vi "DQ_test.vi"() -> ()   [LabVIEW 2015]
uses:
  <vilib>/Analysis/NI_AALBase.lvlib
  AlphaBetaAndDQ_variants/DQtoABC_PowerInvariant_src.vi
  AlphaBetaAndDQ_variants/DQtoABC_noSine_PowerInvariant_src.vi
  AlphaBetaAndDQ_variants/ABCtoDQ_3PhasePowerInvariant_src.vi
  AlphaBetaAndDQ_variants/ABCtoDQ_noSine_2PhasePowerInvariant_src.vi
  AlphaBetaAndDQ_variants/ABCtoDQ_noSine_3PhasePowerInvariant_src.vi
  AlphaBetaAndDQ_variants/ABCtoDQ_2PhasePowerInvariant_src.vi
  AlphaBetaAndDQ_variants/ABCtoDQ_2PhaseUnitaryMagnitude_src.vi
  AlphaBetaAndDQ_variants/DQtoABC_UnitaryMagnitude_src.vi
  AlphaBetaAndDQ_variants/ABCtoDQ_3PhaseUnitaryMagnitude_src.vi
  AlphaBetaAndDQ_variants/ABCtoDQ_noSine_2PhaseUnitaryMagnitude_src.vi
  AlphaBetaAndDQ_variants/DQtoABC_noSine_UnitaryMagnitude_src.vi
  AlphaBetaAndDQ_variants/ABCtoDQ_noSine_3PhaseUnitaryMagnitude_src.vi
  <vilib>/addons/E-Motor Simulation/Utility/NI_EMSim_Utility.lvlib
panel:
  out "2 phase UM error (no sine) stddev":dbl format="%0.2f"
  out "2 phase UM (no Sine) error max":dbl
  out "2 phase UM (no sine) error mean":dbl format="%0.2f"
  out "3phase UM (no sine)error stddev":dbl format="%0.2f"
  out "3 phase UM (no sine) error max":dbl
  out "3 phase UM (no sine) error mean":dbl format="%0.2f"
  out "3 phase UM error stddev":dbl format="%0.2f"
  out "2 phase UM error stddev":dbl format="%0.2f"
  out "3 phase UM error max":dbl
  out "3 phase UM error mean":dbl format="%0.2f"
  out "2 phase UM error max":dbl
  out "2 phase UM error mean":dbl format="%0.2f"
  out "transposed array":sgl[][](graph)
  out "2 phase PI (no sine) error mean":dbl format="%0.2f"
  out "2 phase PI (no Sine) error max":dbl
  out "2 phase PI error (no sine) stddev":dbl format="%0.2f"
  out "3 phase PI (no sine) error mean":dbl format="%0.2f"
  out "3 phase PI (no sine) error max":dbl
  out "3phase PI (no sine)error stddev":dbl format="%0.2f"
  out "3 phase PI error stddev":dbl format="%0.2f"
  out "2 phase PI error stddev":dbl format="%0.2f"
  in  "Imbalance (percent)":dbl
  in  "GridImbalance":bool
  in  "InjectAdditiveNoise":bool
  in  "Noise Magnitude (percent)":dbl
  in  "Magnitude":dbl=1.0
  out "3 phase PI error max":dbl
  out "3 phase PI error mean":dbl format="%0.2f"
  out "2 phase PI error max":dbl
  out "2 phase PI error mean":dbl format="%0.2f"
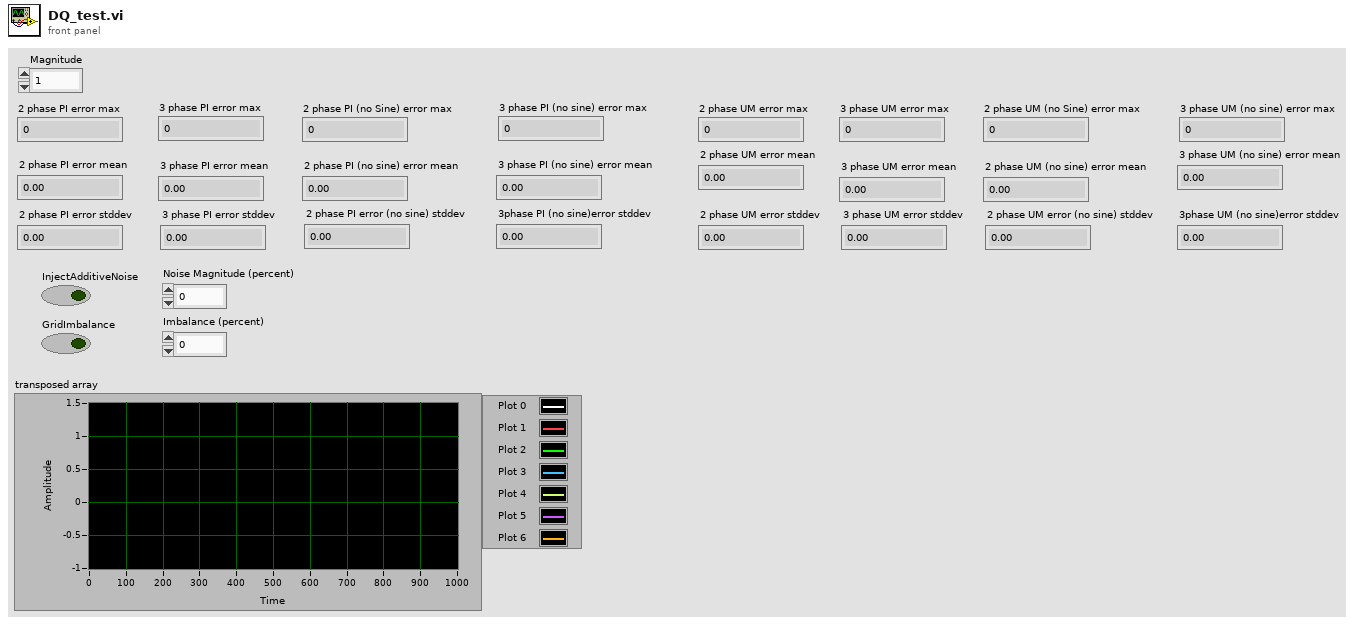
[diagram p1: front panel]
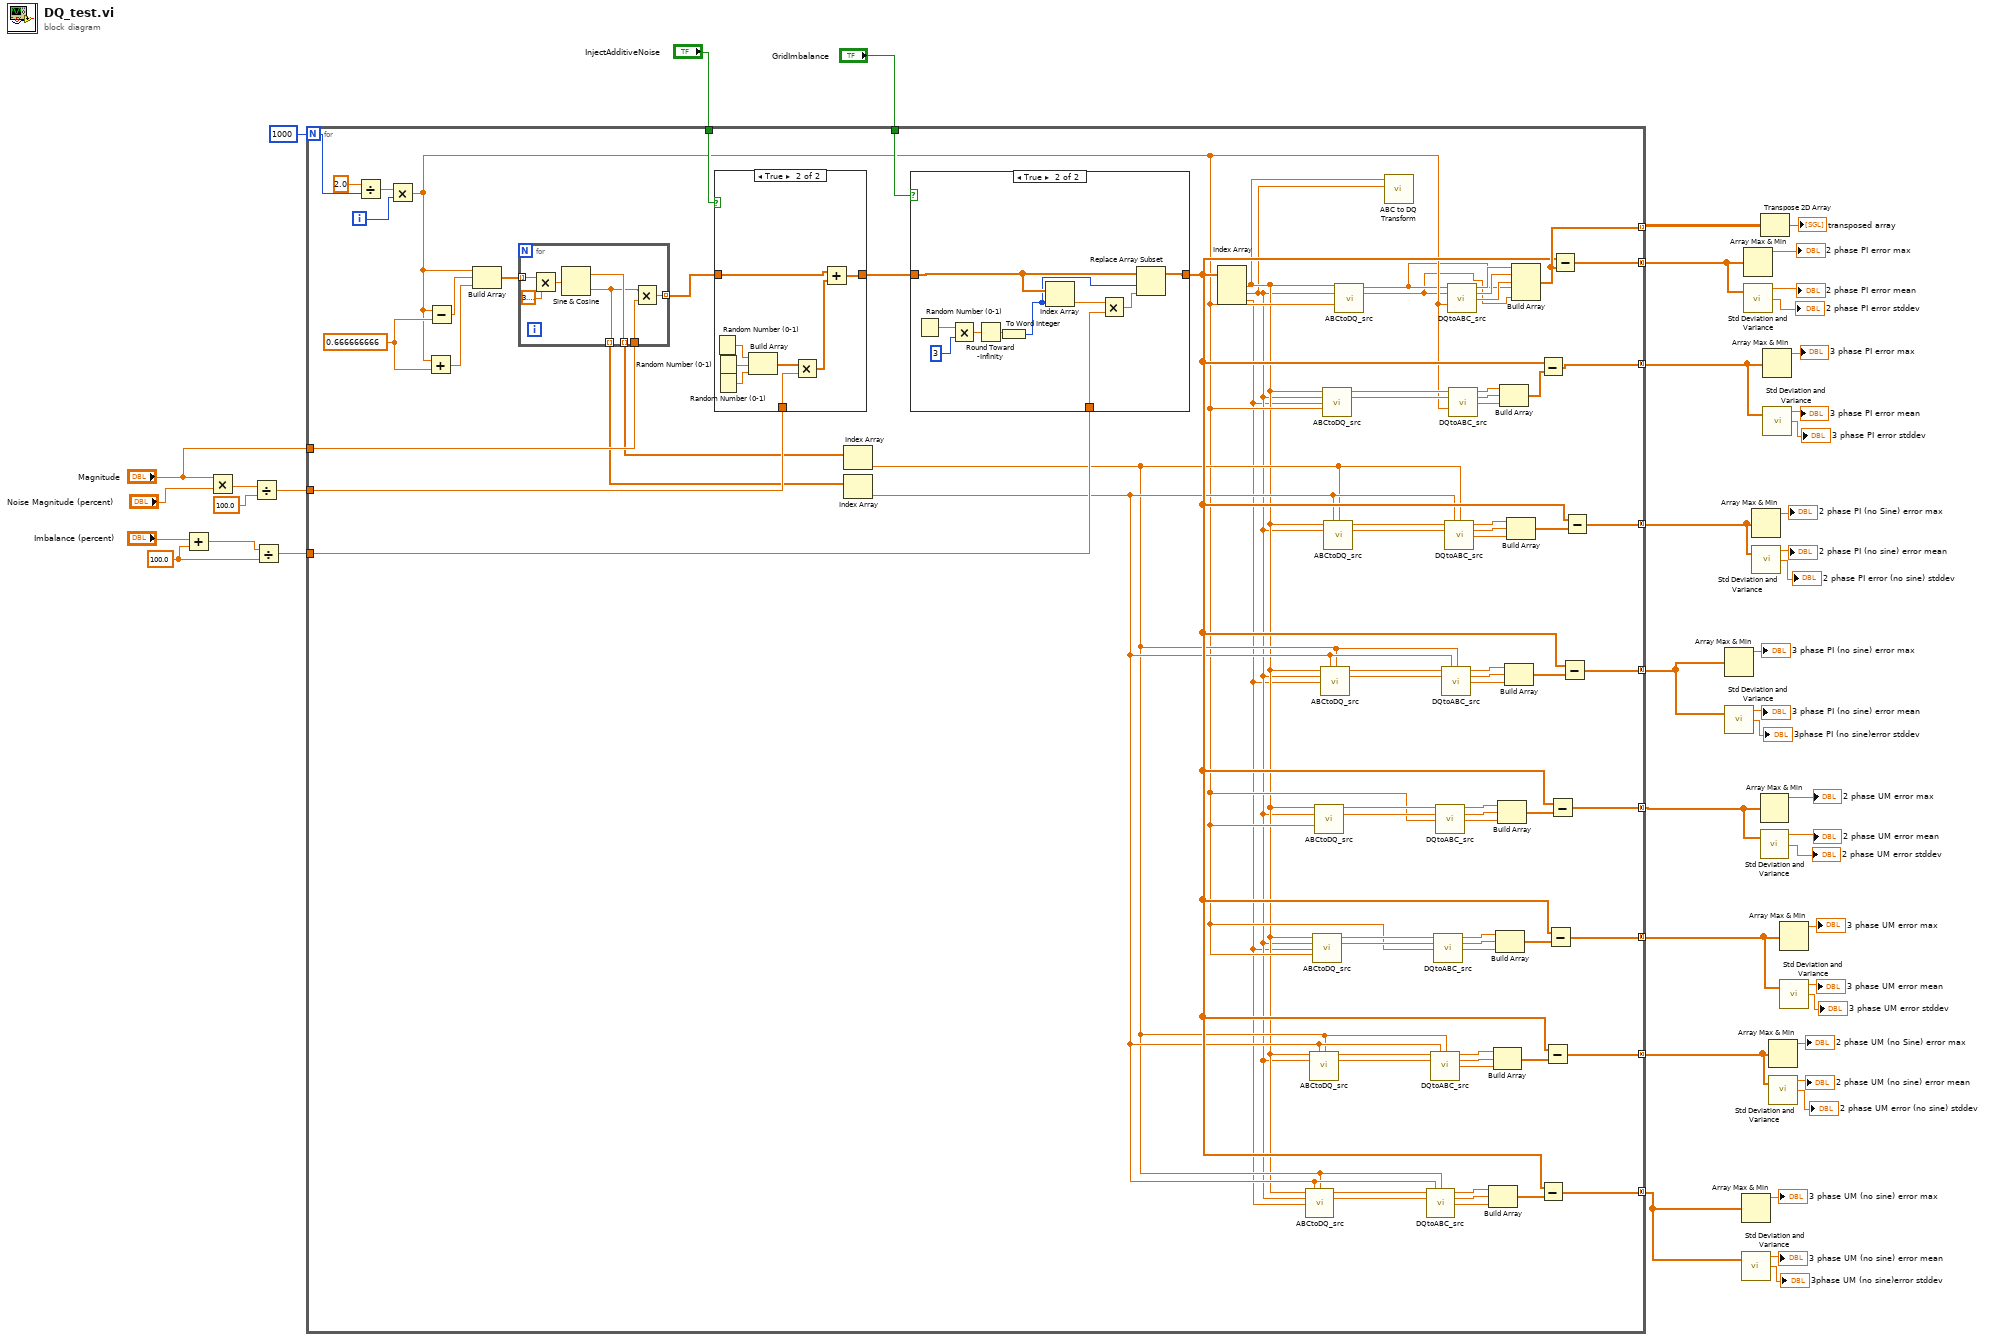
[diagram p0: block diagram]
diagram:
  w31 = 100.0 ("y")
  n1 = Add(x="Imbalance (percent)", y=w31) -> (x+y=w32:dbl)
  n2 = Multiply(x="Magnitude", y="Noise Magnitude (percent)") -> (x*y=w39:dbl)
  n3 = Divide(x=w39, y=100.0) -> (x/y=w36:dbl)
  n4 = Divide(x=w32, y=w31) -> (x/y=w30:dbl)
  n5 = for {
    N: 1000 -> [w115]
    tunnel: [w112] -> w43 mode=concatenating
    tunnel: [w95] -> w19 mode=concatenating
    tunnel: "Magnitude" -> [w122]
    tunnel: w36 -> [w121]
    tunnel: "InjectAdditiveNoise" -> [w120]
    tunnel: "GridImbalance" -> [w119]
    tunnel: w30 -> [w117]
    tunnel: [w102] -> w27 mode=concatenating
    tunnel: [w88] -> w20 mode=concatenating
    tunnel: [w85] -> w17 mode=indexing
    tunnel: [w71] -> w4 mode=concatenating
    tunnel: [w55] -> w3 mode=concatenating
    tunnel: [w54] -> w2 mode=concatenating
    tunnel: [w53] -> w1 mode=concatenating
    i -> [w113]
    w126 = 0.666666666
    n6 = Divide(x=2.0, y=w115) -> (x/y=w114:dbl)
    n7 = Multiply(x=w114, y=w113) -> (x*y=w52:dbl)
    n8 = Add(x=w52, y=w126) -> (x+y=w124:dbl)
    n9 = Subtract(x=w52, y=w126) -> (x-y=w123:dbl)
    n10 = Build Array(w52, w123, w124) -> (w125:dbl[])
    n11 = for {
      tunnel: w125 -> [w153] mode=indexing
      tunnel: [w151] -> w84 mode=indexing
      tunnel: w122 -> [w150]
      tunnel: [w148] -> w87 mode=indexing
      tunnel: [w147] -> w86 mode=indexing
      n12 = Multiply(x=w153, y=3.141592653589793) -> (x*y=w149:dbl)
      n13 = Sine & Cosine(0:w149) -> (1:w148:dbl, 2:w147:dbl)
      n14 = Multiply(x=w147, y=w150) -> (x*y=w151:dbl)
    }
    n15 = case shown="True" w120 {
      tunnel: w84 -> [w138 w140]
      tunnel: [w138 w139] -> w118
      tunnel: w121 -> [_ w142]
      frame False {
      }
      frame True {
        n16 = Random Number (0-1)() -> (number: 0 to 1=w145:dbl)
        n17 = Random Number (0-1)() -> (number: 0 to 1=w146:dbl)
        n18 = Random Number (0-1)() -> (number: 0 to 1=w144:dbl)
        n19 = Build Array(w145, w146, w144) -> (w143:dbl[])
        n20 = Multiply(x=w143, y=w142) -> (x*y=w141:dbl[])
        n21 = Add(x=w140, y=w141) -> (x+y=w139:dbl[])
      }
    }
    n22 = Index Array(array=w87) -> (element=w56:dbl)  [unwired: 1 in]
    n23 = Index Array(array=w86) -> (element=w57:dbl)  [unwired: 1 in]
    n24 = case shown="True" w119 {
      tunnel: w118 -> [w127 w131]
      tunnel: w117 -> [_ w132]
      tunnel: [w127 w129] -> w58
      frame False {
      }
      frame True {
        n25 = Random Number (0-1)() -> (number: 0 to 1=w137:dbl)
        n26 = Multiply(x=w137, y=3) -> (x*y=w135:dbl)
        n27 = Round Toward -Infinity(1:w135) -> (0:w134:dbl)
        n28 = To Word Integer(number=w134) -> (16bit integer=w128:i16)
        n29 = Index Array(array=w131, index=w128) -> (element=w133:dbl)
        n30 = Multiply(x=w133, y=w132) -> (x*y=w130:dbl)
        n31 = Replace Array Subset(array=w131, new element=w130, index=w128) -> (w129:dbl[])
      }
    }
    n32 = Index Array(array=w58) -> (element #1=w49:dbl, element #2=w48:dbl, element #3=w47:dbl)  [unwired: 3 in]
    n33 = call-poly "ABCtoDQ_src.vi"("A"=w49, "cosx"=w57, "sinx"=w56, "B"=w48, "C"=w47) -> ("direct"=w64:sgl, "quadrature"=w63:sgl)  [unwired: 7 in, 2 out]
    n34 = call-poly "ABCtoDQ_src.vi"("A"=w49, "cosx"=w57, "sinx"=w56, "B"=w48) -> ("direct"=w65:sgl, "quadrature"=w66:sgl)  [unwired: 8 in, 2 out]
    n35 = call-poly "ABCtoDQ_src.vi"("A"=w49, "B"=w48, "C"=w47, "Theta"=w52) -> ("direct"=w77:sgl, "quadrature"=w76:sgl)  [unwired: 6 in, 4 out]
    n36 = call-poly "ABCtoDQ_src.vi"("A"=w49, "B"=w48, "Theta"=w52) -> ("direct"=w78:sgl, "quadrature"=w79:sgl)  [unwired: 7 in, 4 out]
    n37 = call-poly "ABCtoDQ_src.vi"("A"=w49, "cosx"=w57, "sinx"=w56, "B"=w48, "C"=w47) -> ("direct"=w94:sgl, "quadrature"=w93:sgl)  [unwired: 7 in, 2 out]
    n38 = call-poly "ABCtoDQ_src.vi"("A"=w49, "B"=w48, "C"=w47, "Theta"=w52) -> ("direct"=w107:sgl, "quadrature"=w108:sgl)  [unwired: 6 in, 4 out]
    n39 = call-poly "ABCtoDQ_src.vi"("A"=w49, "cosx"=w57, "sinx"=w56, "B"=w48) -> ("direct"=w101:sgl, "quadrature"=w100:sgl)  [unwired: 8 in, 2 out]
    n40 = call-poly "ABCtoDQ_src.vi"("A"=w49, "B"=w48, "Theta"=w52) -> ("direct"=w51:sgl, "quadrature"=w50:sgl)  [unwired: 7 in, 4 out]
    n41 = call <vilib>:"ABC to DQ Transform.vi"("b"=w48, "a"=w49) -> ()  [unwired: 7 in, 3 out]
    n42 = call-poly "DQtoABC_src.vi"("d"=w64, "cos"=w57, "sin"=w56, "q"=w63) -> ("a"=w62:sgl, "b"=w61:sgl, "c"=w60:sgl)  [unwired: 7 in, 2 out]
    n43 = call-poly "DQtoABC_src.vi"("d"=w65, "cos"=w57, "sin"=w56, "q"=w66) -> ("a"=w67:sgl, "b"=w68:sgl, "c"=w69:sgl)  [unwired: 7 in, 2 out]
    n44 = call-poly "DQtoABC_src.vi"("direct"=w77, "quadrature"=w76, "theta"=w52) -> ("A"=w75:sgl, "B"=w74:sgl, "C"=w73:sgl)  [unwired: 6 in, 4 out]
    n45 = call-poly "DQtoABC_src.vi"("direct"=w78, "quadrature"=w79, "theta"=w52) -> ("A"=w80:sgl, "B"=w81:sgl, "C"=w82:sgl)  [unwired: 6 in, 4 out]
    n46 = call-poly "DQtoABC_src.vi"("direct"=w94, "cosx"=w57, "sinx"=w56, "quadrature"=w93) -> ("A"=w92:sgl, "B"=w91:sgl, "C"=w90:sgl)  [unwired: 7 in, 2 out]
    n47 = call-poly "DQtoABC_src.vi"("direct"=w101, "cosx"=w57, "sinx"=w56, "quadrature"=w100) -> ("A"=w99:sgl, "B"=w98:sgl, "C"=w97:sgl)  [unwired: 7 in, 2 out]
    n48 = call-poly "DQtoABC_src.vi"("direct"=w51, "quadrature"=w50, "theta"=w52) -> ("A"=w111:sgl, "B"=w110:sgl, "C"=w109:sgl)  [unwired: 6 in, 4 out]
    n49 = call-poly "DQtoABC_src.vi"("direct"=w107, "quadrature"=w108, "theta"=w52) -> ("A"=w104:sgl, "B"=w105:sgl, "C"=w106:sgl)  [unwired: 6 in, 4 out]
    n50 = Build Array(w62, w61, w60) -> (w59:sgl[])
    n51 = Build Array(w67, w68, w69) -> (w70:sgl[])
    n52 = Build Array(w75, w74, w73) -> (w72:sgl[])
    n53 = Build Array(w80, w81, w82) -> (w83:sgl[])
    n54 = Build Array(w104, w105, w106) -> (w103:sgl[])
    n55 = Build Array(w92, w91, w90) -> (w89:sgl[])
    n56 = Build Array(w99, w98, w97) -> (w96:sgl[])
    n57 = Build Array(w111, w110, w109, w51, w50) -> (w85:sgl[])
    n58 = Subtract(x=w58, y=w103) -> (x-y=w102:dbl[])
    n59 = Subtract(x=w58, y=w59) -> (x-y=w53:dbl[])
    n60 = Subtract(x=w58, y=w70) -> (x-y=w54:dbl[])
    n61 = Subtract(x=w58, y=w72) -> (x-y=w55:dbl[])
    n62 = Subtract(x=w58, y=w83) -> (x-y=w71:dbl[])
    n63 = Subtract(x=w58, y=w85) -> (x-y=w112:dbl[])
    n64 = Subtract(x=w58, y=w89) -> (x-y=w88:dbl[])
    n65 = Subtract(x=w58, y=w96) -> (x-y=w95:dbl[])
  }
  n66 = Array Max & Min(array=w20) -> (max value=→"3 phase PI (no sine) error max":dbl)  [unwired: 3 out]
  n67 = call <vilib>:"Std Deviation and Variance.vi"("X"=w20) -> ("mean"=→"3 phase PI (no sine) error mean":dbl, "standard deviation"=→"3phase PI (no sine)error stddev":dbl)  [unwired: 1 in, 1 out]
  n68 = Array Max & Min(array=w1) -> (max value=→"3 phase UM (no sine) error max":dbl)  [unwired: 3 out]
  n69 = call <vilib>:"Std Deviation and Variance.vi"("X"=w1) -> ("mean"=→"3 phase UM (no sine) error mean":dbl, "standard deviation"=→"3phase UM (no sine)error stddev":dbl)  [unwired: 1 in, 1 out]
  n70 = Array Max & Min(array=w43) -> (max value=→"2 phase PI error max":dbl)  [unwired: 3 out]
  n71 = call <vilib>:"Std Deviation and Variance.vi"("X"=w43) -> ("mean"=→"2 phase PI error mean":dbl, "standard deviation"=→"2 phase PI error stddev":dbl)  [unwired: 1 in, 1 out]
  n72 = Array Max & Min(array=w19) -> (max value=→"2 phase PI (no Sine) error max":dbl)  [unwired: 3 out]
  n73 = call <vilib>:"Std Deviation and Variance.vi"("X"=w19) -> ("mean"=→"2 phase PI (no sine) error mean":dbl, "standard deviation"=→"2 phase PI error (no sine) stddev":dbl)  [unwired: 1 in, 1 out]
  n74 = Array Max & Min(array=w4) -> (max value=→"2 phase UM error max":dbl)  [unwired: 3 out]
  n75 = call <vilib>:"Std Deviation and Variance.vi"("X"=w4) -> ("mean"=→"2 phase UM error mean":dbl, "standard deviation"=→"2 phase UM error stddev":dbl)  [unwired: 1 in, 1 out]
  n76 = Transpose 2D Array(2D array=w17) -> (transposed array=→"transposed array":sgl[][])
  n77 = Array Max & Min(array=w27) -> (max value=→"3 phase PI error max":dbl)  [unwired: 3 out]
  n78 = call <vilib>:"Std Deviation and Variance.vi"("X"=w27) -> ("mean"=→"3 phase PI error mean":dbl, "standard deviation"=→"3 phase PI error stddev":dbl)  [unwired: 1 in, 1 out]
  n79 = Array Max & Min(array=w2) -> (max value=→"2 phase UM (no Sine) error max":dbl)  [unwired: 3 out]
  n80 = call <vilib>:"Std Deviation and Variance.vi"("X"=w2) -> ("mean"=→"2 phase UM (no sine) error mean":dbl, "standard deviation"=→"2 phase UM error (no sine) stddev":dbl)  [unwired: 1 in, 1 out]
  n81 = Array Max & Min(array=w3) -> (max value=→"3 phase UM error max":dbl)  [unwired: 3 out]
  n82 = call <vilib>:"Std Deviation and Variance.vi"("X"=w3) -> ("mean"=→"3 phase UM error mean":dbl, "standard deviation"=→"3 phase UM error stddev":dbl)  [unwired: 1 in, 1 out]
